vi "Setup H5 File.vi"(5 "Gyro range (deg/s)":dbl, 6 "block size":i32=100, 7 "Accel range (g)":dbl, 8 "error in (no error)":errorcluster, 10 "Sampling rate (Hz)":dbl, 11 "path in":path) -> (0 "error out":errorcluster, 3 "H5refs":T1 {"File ref" format="%.0x"})   [LabVIEW 2013]
uses:
  H5refs.ctl
  <vilib>/addons/h5labview2/base/hid_t.ctl
  <vilib>/addons/h5labview2/file/H5Fmode.ctl
  <vilib>/addons/h5labview2/base/lib_path.vi
  h5logger/Create HDF5 chunked dataset (1D).vi
  h5logger/Create HDF5 chunked dataset (2D).vi
  <vilib>/addons/h5labview2/base/H5Equery.vi
  <vilib>/addons/h5labview2/attrib/H5Awrite.llb/H5Awrite.xnode
  <vilib>/addons/h5labview2/file/H5F.lvlib
  <vilib>/addons/h5labview2/group/H5G.lvlib
  h5logger/h5logger.lvlib
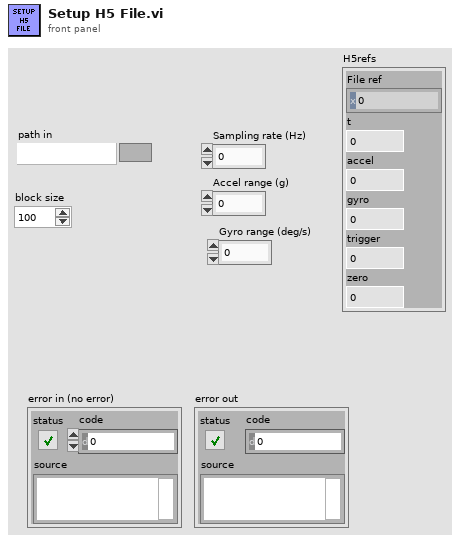
[diagram p1: front panel]
types:
  T1 = typedef "H5refs.ctl" = cluster{"File ref":T2, "t":i32, "accel":i32, "gyro":i32, "trigger":i32, "zero":i32}
  T2 = typedef "hid_t.ctl" = i32
  T3 = typedef "H5F.lvlib/H5Fmode.ctl" = enum16{"read-only", "read-write", "overwrite", "create new", "open or create"}
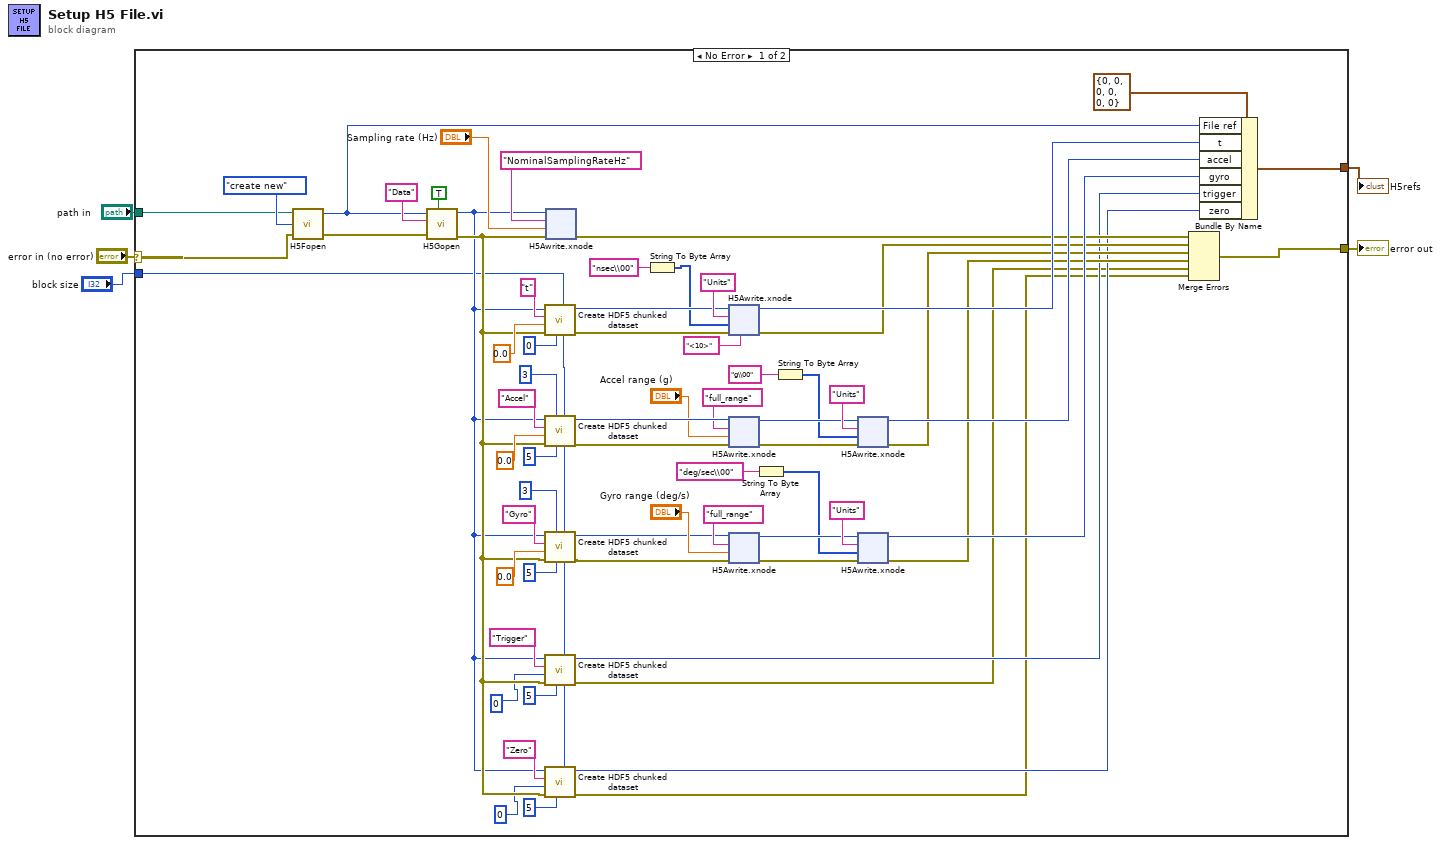
[diagram p0: block diagram]
diagram:
  n1 = case shown="No Error" "error in (no error)" {
    selector: "error in (no error)" -> [w70 w181]
    tunnel: "path in" -> [w71 _]
    tunnel: [w27 w181] -> w2
    tunnel: [w26 _] -> w3
    tunnel: "block size" -> [w6 _]
    frame No Error {
      n2 = call <vilib>:"H5Fopen.vi"("error in (no error)"=w70, "mode (read-only)"=H5Fmode."create new", "path"=w71) -> ("error out"=w69:errorcluster, "ref out"=w25:T2)  [unwired: 1 in]
      n3 = call <vilib>:"H5Gopen.vi"("create? (F)"=TRUE, "error in (no error)"=w69, "name"="Data", "ref in"=w25) -> ("error out"=w19:errorcluster, "group out"=w18:T2)  [unwired: 3 in]
      n4 = call-poly "Create HDF5 chunked dataset.vi"("block size"=w6, "compression"=0, "error in (no error)"=w19, "data type"=0.0, "name"="t", "ref in"=w18) -> ("error out"=w43:errorcluster, "dset out"=w44:i32)  [unwired: 4 in]
      n5 = call-poly "Create HDF5 chunked dataset.vi"("block size"=w6, "compression"=5, "number of channels"=3, "error in (no error)"=w19, "data type"=0.0, "name"="Accel", "ref in"=w18) -> ("error out"=w50:errorcluster, "dset out"=w53:i32)  [unwired: 3 in]
      n6 = call-poly "Create HDF5 chunked dataset.vi"("block size"=w6, "compression"=5, "number of channels"=3, "error in (no error)"=w19, "data type"=0.0, "name"="Gyro", "ref in"=w18) -> ("error out"=w46:errorcluster, "dset out"=w47:i32)  [unwired: 3 in]
      n7 = call-poly "Create HDF5 chunked dataset.vi"("block size"=w6, "compression"=5, "error in (no error)"=w19, "data type"=u8 0 ("compression"), "name"="Trigger", "ref in"=w18) -> ("error out"=w15:errorcluster, "dset out"=w17:i32)  [unwired: 4 in]
      n8 = call-poly "Create HDF5 chunked dataset.vi"("block size"=w6, "compression"=5, "error in (no error)"=w19, "data type"=u8 0 ("compression"), "name"="Zero", "ref in"=w18) -> ("error out"=w14:errorcluster, "dset out"=w16:i32)  [unwired: 4 in]
      n9 = xnode "H5Awrite.xnode"("error in (no error)"=w19, "data"="Sampling rate (Hz)", "attrib name"="NominalSamplingRateHz", "ref in"=w18) -> ("error out"=w31:errorcluster)  [unwired: 3 in, 2 out]
      n10 = String To Byte Array(string="nsec\\00" ("attrib name")) -> (unsigned byte array=w11:u8[])
      n11 = xnode "H5Awrite.xnode"("type name (default)"="<10>", "error in (no error)"=w43, "data"=w11, "attrib name"="Units", "ref in"=w44) -> ("error out"=w30:errorcluster, "ref out"=w34:T2)  [unwired: 2 in, 1 out]
      n12 = xnode "H5Awrite.xnode"("error in (no error)"=w50, "data"="Accel range (g)", "attrib name"="full_range", "ref in"=w53) -> ("error out"=w39:errorcluster, "ref out"=w40:T2)  [unwired: 3 in, 1 out]
      n13 = xnode "H5Awrite.xnode"("error in (no error)"=w46, "data"="Gyro range (deg/s)", "attrib name"="full_range", "ref in"=w47) -> ("error out"=w35:errorcluster, "ref out"=w36:T2)  [unwired: 3 in, 1 out]
      n14 = String To Byte Array(string="deg/sec\\00" ("attrib name")) -> (unsigned byte array=w9:u8[])
      n15 = String To Byte Array(string="g\\00" ("attrib name")) -> (unsigned byte array=w10:u8[])
      n16 = xnode "H5Awrite.xnode"("error in (no error)"=w39, "data"=w10, "attrib name"="Units", "ref in"=w40) -> ("error out"=w29:errorcluster, "ref out"=w33:T2)  [unwired: 3 in, 1 out]
      n17 = xnode "H5Awrite.xnode"("error in (no error)"=w35, "data"=w9, "attrib name"="Units", "ref in"=w36) -> ("error out"=w28:errorcluster, "ref out"=w32:T2)  [unwired: 3 in, 1 out]
      n18 = Merge Errors(w31, w30, w29, w28, w15, w14) -> (w27:errorcluster)
      n19 = Bundle By Name(cluster=T1 {"File ref"=0, "t"=0, "accel"=0, "gyro"=0, "trigger"=0, "zero"=0} ("H5refs"), "File ref"=w25, "t"=w34, "accel"=w33, "gyro"=w32, "trigger"=w17, "zero"=w16) -> (w26:T1)
    }
    frame Error {
    }
  }
  "H5refs" <- w3
  "error out" <- w2
